vi "Threshold Gate.vi"(9 "Value":dbl, 10 "Threshold":dbl=0.01) -> (2 "Output":dbl)   [LabVIEW 2012]
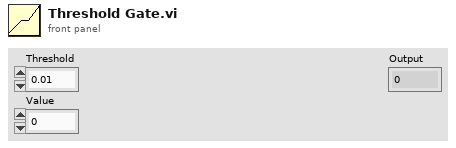
[diagram p1: front panel]
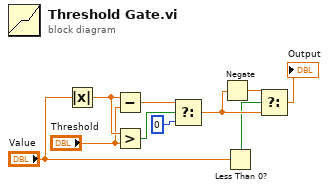
[diagram p0: block diagram]
diagram:
  n1 = Absolute Value(x="Value") -> (abs(x)=w7:dbl)
  n2 = Subtract(x=w7, y="Threshold") -> (x-y=w5:dbl)
  n3 = Greater?(x=w7, y="Threshold") -> (0:w6:bool)
  n4 = Select(t=w5, s=w6, f=0) -> (s? t:f=w9:dbl)
  n5 = Negate(x=w9) -> (-x=w10:dbl)
  n6 = Less Than 0?(x="Value") -> (x < 0?=w8:bool)
  n7 = Select(t=w10, s=w8, f=w9) -> (s? t:f=→"Output":dbl)
